vi "Create and Start gRPC Server.vi"(5 "Server Key File (.key)":path, 7 "Server Certificate File (.crt)":path, 8 "error in (no error)":errorcluster, 11 "CIFTemplateNode in":refnum<class "CIFCorePlugin.lvclass">) -> (0 "error out":errorcluster, 3 "CIFTemplateNode out":refnum<class "CIFCorePlugin.lvclass">)   [LabVIEW 2021, in "CIFCorePlugin.lvclass"]
uses:
  CIFCorePlugin.lvclass
  <vilib>/gRPC/LabVIEW gRPC Servicer/Servicer/Servicer.lvclass/Servicer.ctl
  CIFCorePlugin.lvclass/CIFCorePlugin.ctl
  <vilib>/gRPC/LabVIEW gRPC Servicer/Servicer/Servicer.lvclass
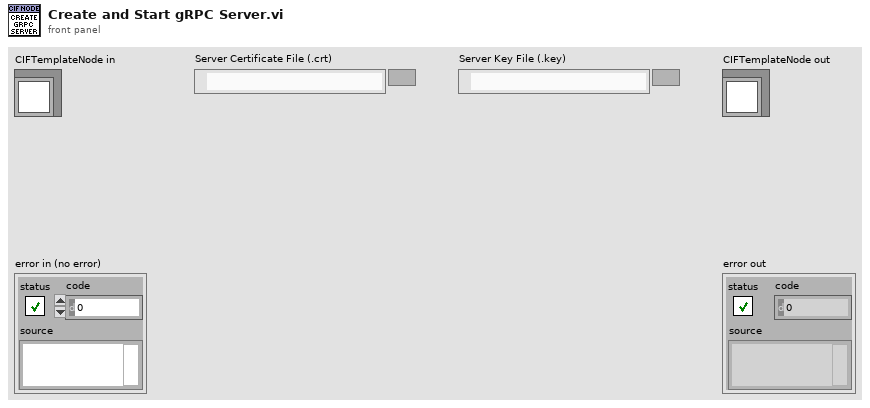
[diagram p1: front panel]
types:
  T1 = typedef "grpc-lvsupport-release.lvlib/grpcId.ctl" = u64
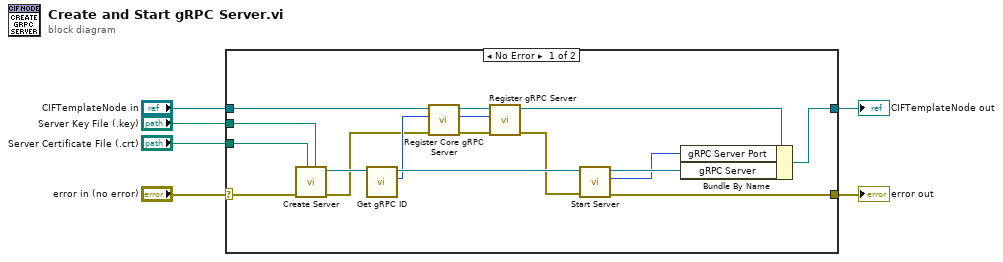
[diagram p0: block diagram]
diagram:
  n1 = case shown="No Error" "error in (no error)" {
    selector: "error in (no error)" -> [w19 w25]
    tunnel: [w11 w25] -> w5
    tunnel: [w7 w24] -> w3
    tunnel: "CIFTemplateNode in" -> [w18 w24]
    tunnel: "Server Certificate File (.crt)" -> [w21 _]
    tunnel: "Server Key File (.key)" -> [w20 _]
    frame No Error {
      n2 = call <vilib>:"Create Server.vi"("Server Key File (.key)"=w20, "Server Certificate File (.crt)"=w21, "error in"=w19) -> ("error out"=w16:errorcluster, "gRPC Server out"=w23:refnum<class "Servicer.lvclass">)  [unwired: 7 in]
      n3 = call <vilib>:"Get gRPC ID.vi"("OOP Server in"=w23) -> ("gRPC ID"=w17:T1, "OOP Server out"=w22:refnum<class "Servicer.lvclass">)  [unwired: 9 in]
      n4 = call "Register Core gRPC Server.vi"("error in (no error)"=w16, "gRPC ID"=w17, "CIFTemplateNode in"=w18) -> ("error out"=w13:errorcluster, "gRPC ID Out"=w14:T1, "CIFTemplateNode out"=w15:refnum<class "CIFCorePlugin.lvclass">)  [unwired: 6 in]
      n5 = call-dynamic "Register gRPC Server.vi"("error in (no error)"=w13, "gRPC ID"=w14, "CIFTemplateNode in"=w15) -> ("error out"=w12:errorcluster, "CIFTemplateNode out"=w10:refnum<class "CIFCorePlugin.lvclass">)  [unwired: 6 in, 1 out]
      n6 = call <vilib>:"Start Server.vi"("error in"=w12, "gRPC Server in"=w22) -> ("error out"=w11:errorcluster, "Listening Port"=w8:i32, "gRPC Server out"=w9:refnum<class "Servicer.lvclass">)  [unwired: 7 in]
      n7 = Bundle By Name(cluster=w10, "gRPC Server Port"=w8, "gRPC Server"=w9) -> (w7:refnum<class "CIFCorePlugin.lvclass">)
    }
    frame Error {
    }
  }
  "error out" <- w5
  "CIFTemplateNode out" <- w3
